vi "TestAFM_Driver_Manager.vi"   [LabVIEW 2020, in "AFM_Driver_Manager.lvclass"]
uses:
  lvsrc/subVIs/AFM API/AFM_Driver_Manager/AFM_Driver_Manager.lvclass
  <userlib>/LevyLab/Relay Box/Type_defs/Resistor--enum.ctl
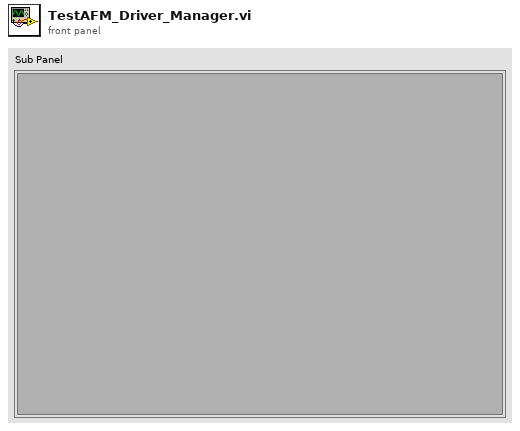
[diagram p1: front panel]
types:
  T1 = typedef "Resistor--enum.ctl" = enum16{"open", "discharge tip", "0 ohms", "100k ohm", "10M ohm", "1G ohm"}
  T2 = cluster{"Name":string, "Litho":cluster{"X":dbl, "Y":dbl, "Speed":dbl, "Voltage":dbl}[], "Set Resistance":T1}[]
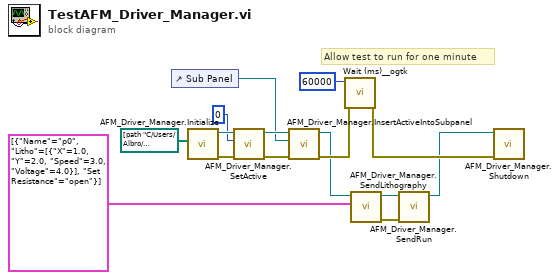
[diagram p0: block diagram]
diagram:
  # "Allow test to run for one minute"
  n1 = control-ref of="Sub Panel"() -> (w10:refnum<vi>)
  n2 = call "AFM_Driver_Manager.Initialize.vi"("Paths"=path[] [path "C:/Users/Albro/Documents/GitHub/AFM-Lithography/lvsrc/AFMs/Asylum_Driver/Asylum_Driver.vi"]) -> ("error out"=w14:errorcluster, "AFM_Driver_Manager out"=w15:refnum<class "AFM_Driver_Manager.lvclass">)  [unwired: 9 in]
  n3 = call "AFM_Driver_Manager.SetActive.vi"("error in (no error)"=w14, "Active Index"=0, "AFM_Driver_Manager in"=w15) -> ("error out"=w12:errorcluster, "AFM_Driver_Manager out"=w13:refnum<class "AFM_Driver_Manager.lvclass">)  [unwired: 7 in]
  n4 = call "AFM_Driver_Manager.InsertActiveIntoSubpanel.vi"("error in (no error)"=w12, "SubPnl Refnum"=w10, "AFM_Driver_Manager in"=w13) -> ("error out"=w8:errorcluster, "AFM_Driver_Manager out"=w2:refnum<class "AFM_Driver_Manager.lvclass">)  [unwired: 7 in]
  n5 = call <userlib>:"Wait (ms)__ogtk.vi"("error in (no error)"=w8, "milliseconds to wait"=u32 60000) -> ("error out"=w3:errorcluster)  [unwired: 8 in, 1 out]
  n6 = call "AFM_Driver_Manager.SendLithography.vi"("Lithography Data"=T2 [{"Name"="p0", "Litho"=[{"X"=1.0, "Y"=2.0, "Speed"=3.0, "Voltage"=4.0}], "Set Resistance"=enum."open"}], "AFM_Driver_Manager in"=w2) -> ("error out"=w4:errorcluster, "AFM_Driver_Manager out"=w5:refnum<class "AFM_Driver_Manager.lvclass">)  [unwired: 8 in]
  n7 = call "AFM_Driver_Manager.SendRun.vi"("error in (no error)"=w4, "AFM_Driver_Manager in"=w5) -> ("AFM_Driver_Manager out"=w1:refnum<class "AFM_Driver_Manager.lvclass">)  [unwired: 8 in, 1 out]
  n8 = call "AFM_Driver_Manager.Shutdown.vi"("error in (no error)"=w3, "AFM_Driver_Manager in"=w1) -> ()  [unwired: 8 in, 2 out]
